vi "Get Setpoint.vi"(8 "error in (no error)":errorcluster, 11 "Alicat Controller in":refnum<class "Alicat Controller.lvclass">) -> (0 "error out":errorcluster, 2 "Setpoint":sgl, 3 "Alicat Controller out":refnum<class "Alicat Controller.lvclass">)   [LabVIEW 2014, in "Alicat.lvlib" / "Alicat Controller.lvclass"]
uses:
  Alicat Controller.lvclass
  Alicat Controller.lvclass/Alicat Controller.ctl
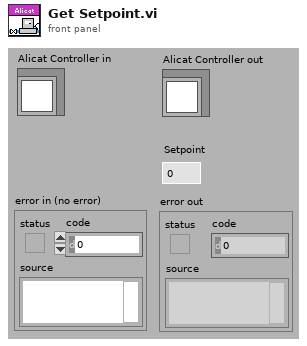
[diagram p1: front panel]
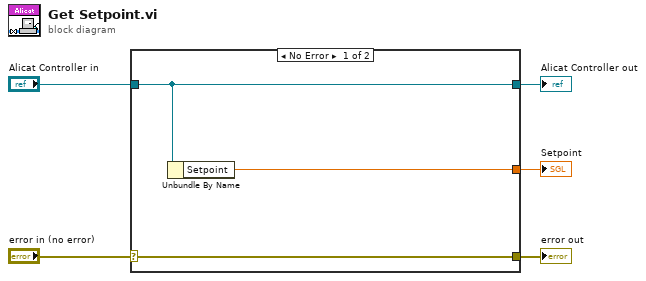
[diagram p0: block diagram]
diagram:
  n1 = case shown="No Error" "error in (no error)" {
    selector: "error in (no error)" -> [w8 w9]
    tunnel: [w8 w9] -> w4
    tunnel: [w7 w10] -> w2
    tunnel: "Alicat Controller in" -> [w7 w10]
    tunnel: [w6 _] -> w1
    frame No Error {
      n2 = Unbundle By Name(w7) -> ("Setpoint"=w6:sgl)
    }
    frame Error {
    }
  }
  "error out" <- w4
  "Alicat Controller out" <- w2
  "Setpoint" <- w1
